vi "Main v1.1.vi"() -> ()   [LabVIEW 2017]
doc: "v0.85:\n- Counts for rejects and total\n\nv0.5:\n\n- Added Reject to Manual Mode\n- Send reject pallet cluster during manual mode\n- Run continuous manual happens only when no error has occured"
uses:
  Controls/Main Tabs v0.1.ctl
  Controls/Auto.ctl
  RT/Controls/Auto Delays.ctl
  RT/Controls/Auto Times.ctl
  support/Controls/General Para.ctl
  Controls/UI Data.ctl
  support/Controls/Auto Stats.ctl
  Controls/Logging FGV.ctl
  support/Message Queue/Enqueue Message (Single).vi
  GV/Maintenance GV.vi
  <vilib>/Utility/error.llb/Error Cluster From Error Code.vi
  <vilib>/ErrorRing/Error Ring.xnode
  support/Message Queue/Message Queue.lvlib
  support/User Event - Stop/User Event - Stop.lvlib
panel:
  in  "General Para 2":T1={"Max. Cons."=5.0, "Offset 1"=0.0, "Offset 2"=0.0, "Offset 3"=0.0, "Offset 4"=0.0} caption="General Para"
  in  "Auto Para 2":T2={"Agitator Delays"=[250, 350], "TF Delays"=[700, 800, 2], "Insertion Delays"=[100, 500], "Cutting Delays"=[300, 300, 100], "PF Delays"=[250, 30000], "Measur. Delays"=[500.0, 188.9, 1.0], "Reject Delays"=[500], "BF Delays"=[1000, 1000]}
  out "Shutdown?":bool
  out "Boolean 8":bool
  out "Boolean 7":bool
  out "Boolean 6":bool
  out "Boolean 5":bool
  out "Boolean 4":bool
  out "Boolean 3":bool
  out "Boolean 2":bool
  out "Boolean":bool
  in  "Reject Pallets":T3
  out "Date-Time":string caption="Dip-Tube Assembly Automation (HMI) v1.1"
  out "Main Tab":T4
  in  "All IOs":bool
  in  "Autocycle":T5
  in  "Manual":bool
  in  "Parameters":bool
  in  "Maintenance":bool
  in  "General Para":T1={"Max. Cons."=5.0, "Offset 1"=0.0, "Offset 2"=0.0, "Offset 3"=0.0, "Offset 4"=0.0}
  in  "BF Para":cluster{"Delay 1":u32, "Delay 2":u32}={"Delay 1"=1000, "Delay 2"=1000}
  in  "Reject Para":cluster{"Delay":u32}={"Delay"=400}
  in  "Meas. Para":T6={"Delay"=500.0, "Mean Length"=188.9, "Tolerance"=1.0}
  in  "PF Para":cluster{"Delay":u32, "Timeout":u32}={"Delay"=1000, "Timeout"=1000}
  in  "Tube Feeder Para":T7={"Delay"=400, "Delay 2"=250, "Max Attempts"=250}
  in  "Cutting Para":T8={"Delay"=400, "Delay 2"=250, "Delay 3"=250}
  in  "Agitator Para":cluster{"Delay":u32, "Timeout":u32}={"Delay"=400, "Timeout"=250}
  in  "Insertion Para":cluster{"Delay 1":u32, "Delay 2":u32}={"Delay 1"=1000, "Delay 2"=1000}
  in  "Save Para":bool
  in  "Home Para":bool
  out "OEE":dbl format="%#.1f"
  out "QUA":dbl=100.0 min=0.0 max=100.0 step=0.1
  in  "Ideal Time":dbl=2.0 min=0.0 max=100.0 step=0.1
  in  "AVL":dbl=100.0 min=0.0 max=100.0 step=0.1
  out "Rejects 2":u32 caption="Rejects"
  in  "Reset MCount":bool
  in  "Enable BF?":bool
  in  "Enable Agitate?":bool
  in  "Enable Reject?":bool
  in  "Toggle Motor":bool
  in  "Continuous?":bool
  in  "Enable Measure?":bool
  in  "Enable Index?":bool
  in  "Enable PF?":bool
  in  "Manual Para":T2={"Agitator Delays"=[400, 250], "TF Delays"=[700, 800, 2], "Insertion Delays"=[100, 500], "Cutting Delays"=[300, 300, 100], "PF Delays"=[250, 30000], "Measur. Delays"=[500.0, 188.9, 1.0], "Reject Delays"=[500], "BF Delays"=[1000, 1000]}
  in  "Enable Cutting?":bool
  in  "Enable Insertion?":bool
  in  "Run Manual":bool
  in  "Enable TF?":bool
  in  "Home Manual":bool
  out "Status 2":T10
  out "Measurements":T11 {"Height 1" format="%#.2f"; "Height 2" format="%#.2f"; "Height 3" format="%#.2f"; "Height 4" format="%#.2f"}
  out "Output Count":u32 caption="Output\nCount"
  out "PRF":dbl=100.0 min=0.0 max=100.0 step=0.1
  in  "End Cycle":bool
  out "Statuses":string[][](table)
  in  "All IO":bool
  in  "Stats":bool
  in  "Home AC":bool
  out "Status":string
  out "Count":u32 format="%06.0f"
  out "Cycle Time":dbl format="%0.2f"
  out "Rejects":u32 format="%06.0f"
  out "Output Chart":T12(graph)
  out "Reject Count":u32
  out "Total Count":u32 caption="Good Count"
  out "Total Time":dbl caption="Total Effective Cycle Time (s)" format="%#.3f"
  out "Time Chart":T13(graph)
  out "OEE Chart":T14(graph)
  out "Measurement Chart":cluster{"1":dbl, "2":dbl, "3":dbl, "4":dbl}(graph)
  out "Timestamp":string caption="Date & Timestamp"
  out "Latest Measure.":T15 caption="Latest Measurements" {"Length 1 (mm)" format="%#.2f"}
  out "Auto Times":T9
  in  "Back Stats":bool
  out "OEE 2":T14 caption="Latest Measurements" {"AVL" format="%#.1f"; "PRF" format="%#.1f"; "QUA" format="%#.1f"; "OEE" format="%#.1f"}
  in  "Home IOs":bool
  in  "Back IO":bool
  out "IAS 4":dbl format="%#.3f"
  out "IAS 3":dbl format="%#.3f"
  out "IAS 2":dbl format="%#.3f"
  out "IAS 1":dbl format="%#.3f"
  out "DI 1":T16
  out "DI 2":T17
  out "DO 1":T18
  in  "Exit":bool
  in  "Shutdown":bool
  # "HARMONY VISION DIP-TUBE ASSEMBLY AUTOMATION"
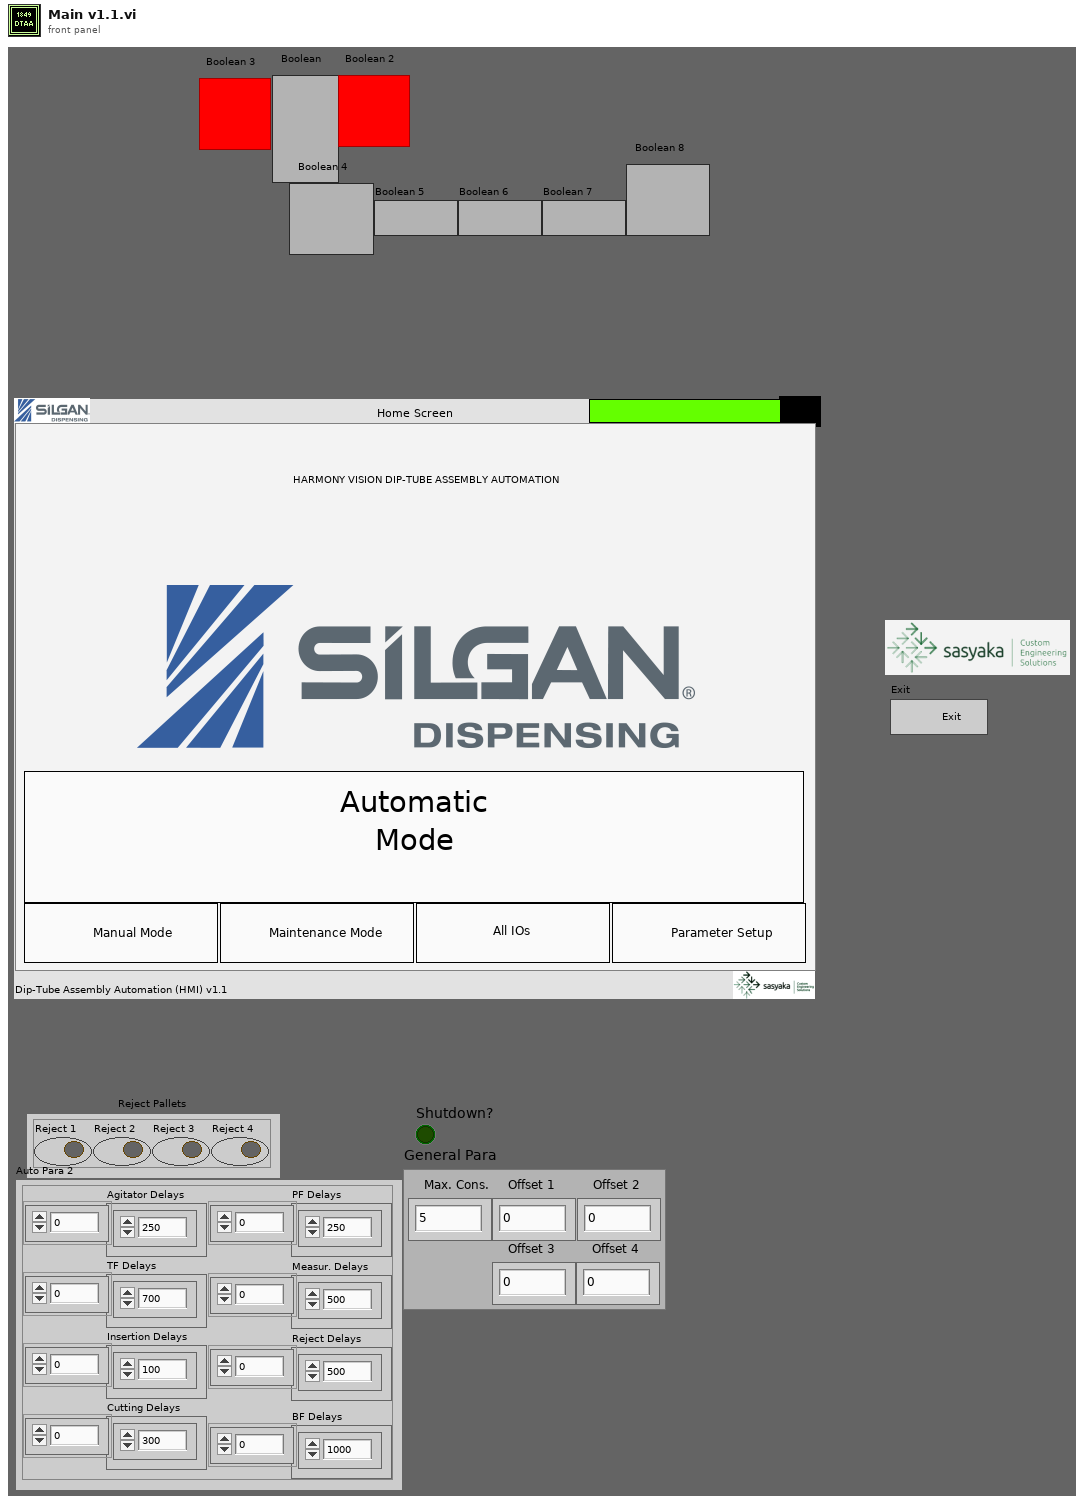
[diagram p1: front panel]
types:
  T1 = typedef "General Para.ctl" = cluster{"Max. Cons.":dbl, "Offset 1":dbl, "Offset 2":dbl, "Offset 3":dbl, "Offset 4":dbl}
  T2 = typedef "Auto Delays.ctl" = cluster{"Agitator Delays":u32[], "TF Delays":u32[], "Insertion Delays":u32[], "Cutting Delays":u32[], "PF Delays":u32[], "Measur. Delays":dbl[], "Reject Delays":u32[], "BF Delays":u32[]}
  T3 = cluster{"Reject 1":bool, "Reject 2":bool, "Reject 3":bool, "Reject 4":bool}
  T4 = typedef "Main Tabs v0.1.ctl" = enum32{"Home Screen", "Parameter Setup", "Manual Mode", "Autocycle", "Autocycle Statistics", "Autocycle IOs"}
  T5 = typedef "Auto.ctl" = bool
  T6 = cluster{"Delay":dbl, "Mean Length":dbl, "Tolerance":dbl}
  T7 = cluster{"Delay":u32, "Delay 2":u32, "Max Attempts":u32}
  T8 = cluster{"Delay":u32, "Delay 2":u32, "Delay 3":u32}
  T9 = typedef "Auto Times.ctl" = cluster{"Index Time":u32, "TF Time":u32, "Insertion Time":u32, "Cutting Time":u32, "PF Time":u32, "Meas. Time":u32, "Reject Time":u32}
  T10 = cluster{"Auto Times":T9, "error out":errorcluster}
  T11 = cluster{"Height 1":dbl, "Height 2":dbl, "Height 3":dbl, "Height 4":dbl}
  T12 = cluster{"OutputCount":u32, "Numeric Control":u32}
  T13 = cluster{"Index":dbl, "TF":dbl, "Insert":dbl, "Cutting":dbl, "PF":dbl, "Measure.":dbl, "Reject":dbl}
  T14 = cluster{"AVL":dbl, "PRF":dbl, "QUA":dbl, "OEE":dbl}
  T15 = cluster{"Length 1 (mm)":dbl, "Pallet 2 (mm)":dbl, "Pallet 3 (mm)":dbl, "Pallet 4 (mm)":dbl}
  T16 = cluster{"Machine_ON":bool, "E_stop ":bool, "SW_Pressure":bool, "SW_Start ":bool, "SW_Reset":bool, "SW_Stop":bool, "SW_Door":bool, "RS_Index_Rotary_CW":bool, "RS_Index_Rotary_CCW":bool, "RS_Index_Stopper _Rear":bool, "RS_Index_Output_Separator_Rear":bool, "PES_Index_Pallet_Sensor":bool, "PES_Index_Output_Part Sensor":bool, "ICS_BF_Low_Level_1":bool, "ICS_BF_Low_Level_2":bool, "ICS_BF_Pump_CNVR_Full_1":bool, "ICS_BF_Pump_CNVR_Full_2":bool, "ICS_BF_Pump_CNVR_Full_3":bool, "ICS_BF_Pump_CNVR_Full_4":bool, "PES_PC_Pump Presence_1":bool, "PES_PC_Pump Presence_2":bool, "PES_PC_Pump Presence_3":bool, "PES_PC_Pump Presence_4":bool, "RS_PC_Gating_Front":bool, "PES_Pump_Interference":bool, "PES_TF_Low_Level":bool, "PES_Tube Presence_1":bool, "PES_Tube Presence_2":bool, "PES_Tube Presence_3":bool, "PES_Tube Presence_4":bool, "DI1.30":bool, "DI1.31":bool}
  T17 = cluster{"RS_Agitatator_1_Rear ":bool, "RS_Agitatator_2_Rear ":bool, "RS_TF_Gating CYL_Rear":bool, "RS_Insertion_1_Rear":bool, "RS_Insertion_1_Front":bool, "RS_Insertion _2_Rear":bool, "RS_Insertion _2_Front":bool, "RS_Insertion _3_Rear":bool, "RS_Insertion _3_Front":bool, "RS_Insertion _4_Rear":bool, "RS_Insertion _4_Front":bool, "RS_Insertion_Clamp_Rear":bool, "RS_Cutting_Rear":bool, "RS_Cutting_Clamp _Rear":bool, "RS_Measurement_1_Rear":bool, "RS_Measurement_2_Rear":bool, "RS_Measurement_3_Rear":bool, "RS_Measurement_4_Rear":bool, "DI2.18":bool, "RS_Rejection_1_Rear":bool, "RS_Rejection_2_Rear":bool, "RS_Rejection_3_Rear":bool, "RS_Rejection_4_Rear":bool, "DI2.23":bool, "DI2.24":bool, "DI2.25":bool, "DI2.26":bool, "DI2.27":bool, "DI2.28":bool, "DI2.29":bool, "DI2.30":bool, "DI2.31":bool}
  T18 = cluster{"TL_Red":bool, "TL_Orange":bool, "TL_Green":bool, "TL_Buzzer":bool, "SOL_Index_Rotary_CW":bool, "SOL_Index_Rotary_CCW":bool, "SOL_Index_Stopper_Rear":bool, "SOL_OutputSeparator_Rear":bool, "Bowl  Feeder_ ON 1":bool, "Pump_CNVR_Motor _ON":bool, "SOL_PC_Gating_CYL_Rear":bool, "SOL_Tube_Feed_Agitatator":bool, "SOL_Tube_Feed_Gating_CYL":bool, "SOL_Insertion _CYL":bool, "SOL_Insertion_Clamp_CYL":bool, "SOL_Cutting_CYL":bool, "SOL_Cutting_Clamp_CYL":bool, "SOL_Insertion_Air_Nozzle":bool, "SOL_Measurement_CYL":bool, "DO1.19":bool, "SOL_Rejection CYL_1":bool, "SOL_Rejection CYL_2":bool, "SOL_Rejection CYL_3":bool, "SOL_Rejection CYL_4":bool, "Bowl  Feeder_ ON 2":bool, "SOL_BF_BlowerON":bool, "SOL_BF1_Track1":bool, "SOL_BF1_Track2":bool, "SOL_BF2_Track1":bool, "SOL_BF2_Track2":bool, "DO1.30":bool, "DO1.31":bool}
  T19 = typedef "UI Data.ctl" = cluster{"Main Tab":refnum<vi>}
  T20 = typedef "Message Queue.lvlib/All Message Queues.ctl" = cluster{"UI":refnum<queue>}
  T21 = enum8{"Enabled", "Disabled", "Disabled and Grayed Out"}
  T22 = cluster{"Array":string[][], "Machine Status":string}
  T23 = typedef "Logging FGV.ctl" = enum16{"Start Shift", "Log Index", "Read Shift", "Close Shift"}
  T24 = typedef "Auto Stats.ctl" = cluster{"Time-Stamp":timestamp, "Auto Times":T9, "Measurements":cluster{"1":dbl, "2":dbl, "3":dbl, "4":dbl}, "Outputs":cluster{"Good Parts":u32, "Reject Parts":u32}, "Cycle Time":dbl, "Remarks":string}
  T25 = cluster{"Auto Times":T9, "Results":cluster{"Measurements":cluster{"1":dbl, "2":dbl, "3":dbl, "4":dbl}, "Reject Pallets":cluster{"Reject 1":bool, "Reject 2":bool, "Reject 3":bool, "Reject 4":bool}}, "OutputCount":u32, "error out":errorcluster}
  T26 = enum8{"Information", "Error", "Successful", "Tips"}
  T27 = cluster{"Agitator Delays[0]":u32, "Agitator Delays[1]":u32}
  T28 = cluster{"TF Delays[0]":u32, "TF Delays[1]":u32, "TF Delays[2]":u32}
  T29 = cluster{"Insertion Delays[0]":u32, "Insertion Delays[1]":u32}
  T30 = cluster{"Cutting Delays[0]":u32, "Cutting Delays[1]":u32, "Cutting Delays[2]":u32}
  T31 = cluster{"Measur. Delays[0]":dbl, "Measur. Delays[1]":dbl, "Measur. Delays[2]":dbl}
  T32 = typedef "All Inputs.ctl" = cluster{"DI 1":cluster{"Machine_ON":bool, "E_stop ":bool, "SW_Pressure":bool, "SW_Start ":bool, "SW_Reset":bool, "SW_Stop":bool, "SW_Door":bool, "RS_Index_Rotary_CW":bool, "RS_Index_Rotary_CCW":bool, "RS_Index_Stopper _Rear":bool, "RS_Index_Output_Separator_Rear":bool, "PES_Index_Pallet_Sensor":bool, "PES_Index_Output_Part Sensor":bool, "ICS_BF_Low_Level_1":bool, "ICS_BF_Low_Level_2":bool, "ICS_BF_Pump_CNVR_Full_1":bool, "ICS_BF_Pump_CNVR_Full_2":bool, "ICS_BF_Pump_CNVR_Full_3":bool, "ICS_BF_Pump_CNVR_Full_4":bool, "PES_PC_Pump Presence_1":bool, "PES_PC_Pump Presence_2":bool, "PES_PC_Pump Presence_3":bool, "PES_PC_Pump Presence_4":bool, "RS_PC_Gating_Front":bool, "PES_Pump_Interference":bool, "PES_TF_Low_Level":bool, "PES_Tube Presence_1":bool, "PES_Tube Presence_2":bool, "PES_Tube Presence_3":bool, "PES_Tube Presence_4":bool, "DI1.30":bool, "DI1.31":bool}, "DI 2":cluster{"RS_Agitatator_1_Rear ":bool, "RS_Agitatator_2_Rear ":bool, "RS_TF_Gating CYL_Rear":bool, "RS_Insertion_1_Rear":bool, "RS_Insertion_1_Front":bool, "RS_Insertion _2_Rear":bool, "RS_Insertion _2_Front":bool, "RS_Insertion _3_Rear":bool, "RS_Insertion _3_Front":bool, "RS_Insertion _4_Rear":bool, "RS_Insertion _4_Front":bool, "RS_Insertion_Clamp_Rear":bool, "RS_Cutting_Rear":bool, "RS_Cutting_Clamp _Rear":bool, "RS_Measurement_1_Rear":bool, "RS_Measurement_2_Rear":bool, "RS_Measurement_3_Rear":bool, "RS_Measurement_4_Rear":bool, "RS_Measure_Clamp_Rear":bool, "RS_Rejection_1_Rear":bool, "RS_Rejection_2_Rear":bool, "RS_Rejection_3_Rear":bool, "RS_Rejection_4_Rear":bool, "DI2.23":bool, "DI2.24":bool, "DI2.25":bool, "DI2.26":bool, "DI2.27":bool, "DI2.28":bool, "DI2.29":bool, "DI2.30":bool, "DI2.31":bool}, "IAS 1":dbl, "IAS 2":dbl, "IAS 3":dbl, "IAS 4":dbl, "DO 1":cluster{"TL_Red":bool, "TL_Orange":bool, "TL_Green":bool, "TL_Buzzer":bool, "SOL_Index_Rotary_CW":bool, "SOL_Index_CNVR_Rotary_CCW":bool, "SOL_Index_CNVR_Stopper_Rear":bool, "SOL_Index_CNVR_Output _Separator _Rear":bool, "Bowl  Feeder_ ON 1":bool, "Pump_CNVR_Motor _ON":bool, "SOL_PC_Gating_CYL_Rear":bool, "SOL_Tube_Feed_Agitatator":bool, "SOL_Tube_Feed_Gating_CYL":bool, "SOL_Insertion _CYL":bool, "SOL_Insertion_Clamp_CYL":bool, "SOL_Cutting_CYL":bool, "SOL_Cutting_Clamp_CYL":bool, "SOL_Insertion_Air_Nozzle":bool, "SOL_Measurement_CYL":bool, "DO1.19":bool, "SOL_Rejection CYL_1":bool, "SOL_Rejection CYL_2":bool, "SOL_Rejection CYL_3":bool, "SOL_Rejection CYL_4":bool, "Bowl  Feeder_ ON 2":bool, "SOL_BF_BlowerON":bool, "SOL_BF1_Track1":bool, "SOL_BF1_Track2":bool, "SOL_BF2_Track1":bool, "SOL_BF2_Track2":bool, "DO1.30":bool, "DO1.31":bool}}
  T33 = cluster{"RS_Agitatator_1_Rear ":bool, "RS_Agitatator_2_Rear ":bool, "RS_TF_Gating CYL_Rear":bool, "RS_Insertion_1_Rear":bool, "RS_Insertion_1_Front":bool, "RS_Insertion _2_Rear":bool, "RS_Insertion _2_Front":bool, "RS_Insertion _3_Rear":bool, "RS_Insertion _3_Front":bool, "RS_Insertion _4_Rear":bool, "RS_Insertion _4_Front":bool, "RS_Insertion_Clamp_Rear":bool, "RS_Cutting_Rear":bool, "RS_Cutting_Clamp _Rear":bool, "RS_Measurement_1_Rear":bool, "RS_Measurement_2_Rear":bool, "RS_Measurement_3_Rear":bool, "RS_Measurement_4_Rear":bool, "RS_Measure_Clamp_Rear":bool, "RS_Rejection_1_Rear":bool, "RS_Rejection_2_Rear":bool, "RS_Rejection_3_Rear":bool, "RS_Rejection_4_Rear":bool, "DI2.23":bool, "DI2.24":bool, "DI2.25":bool, "DI2.26":bool, "DI2.27":bool, "DI2.28":bool, "DI2.29":bool, "DI2.30":bool, "DI2.31":bool}
  T34 = cluster{"TL_Red":bool, "TL_Orange":bool, "TL_Green":bool, "TL_Buzzer":bool, "SOL_Index_Rotary_CW":bool, "SOL_Index_CNVR_Rotary_CCW":bool, "SOL_Index_CNVR_Stopper_Rear":bool, "SOL_Index_CNVR_Output _Separator _Rear":bool, "Bowl  Feeder_ ON 1":bool, "Pump_CNVR_Motor _ON":bool, "SOL_PC_Gating_CYL_Rear":bool, "SOL_Tube_Feed_Agitatator":bool, "SOL_Tube_Feed_Gating_CYL":bool, "SOL_Insertion _CYL":bool, "SOL_Insertion_Clamp_CYL":bool, "SOL_Cutting_CYL":bool, "SOL_Cutting_Clamp_CYL":bool, "SOL_Insertion_Air_Nozzle":bool, "SOL_Measurement_CYL":bool, "DO1.19":bool, "SOL_Rejection CYL_1":bool, "SOL_Rejection CYL_2":bool, "SOL_Rejection CYL_3":bool, "SOL_Rejection CYL_4":bool, "Bowl  Feeder_ ON 2":bool, "SOL_BF_BlowerON":bool, "SOL_BF1_Track1":bool, "SOL_BF1_Track2":bool, "SOL_BF2_Track1":bool, "SOL_BF2_Track2":bool, "DO1.30":bool, "DO1.31":bool}
  T35 = cluster{"Manual Para":T2, "Reject Pallets":cluster{"Reject 1":bool, "Reject 2":bool, "Reject 3":bool, "Reject 4":bool}}
  T36 = cluster{"Measurements":cluster{"1":dbl, "2":dbl, "3":dbl, "4":dbl}, "Reject Pallets":cluster{"Reject 1":bool, "Reject 2":bool, "Reject 3":bool, "Reject 4":bool}}
  T37 = cluster{"Reject Pallets":cluster{"Reject 1":bool, "Reject 2":bool, "Reject 3":bool, "Reject 4":bool}, "Measurements":cluster{"1":dbl, "2":dbl, "3":dbl, "4":dbl}}
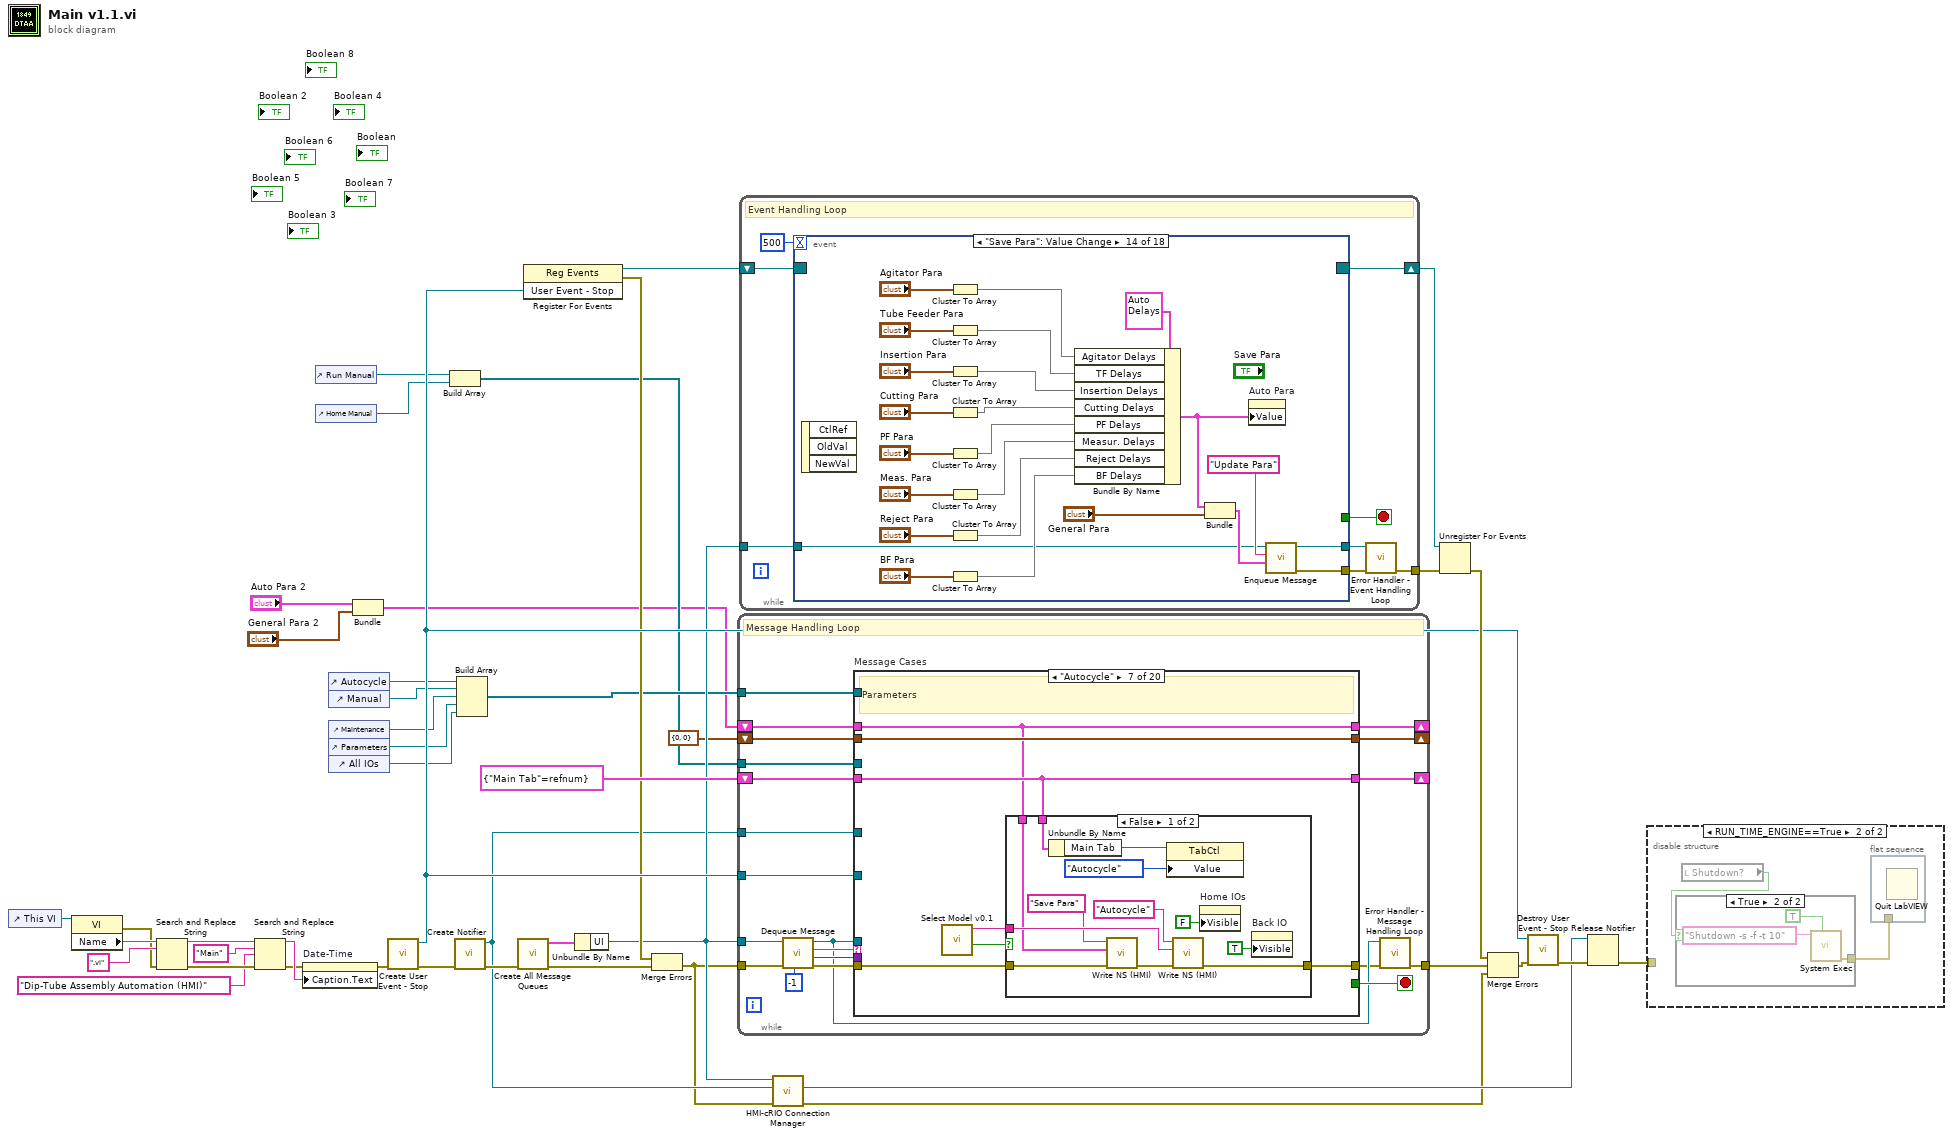
[diagram p0: block diagram]
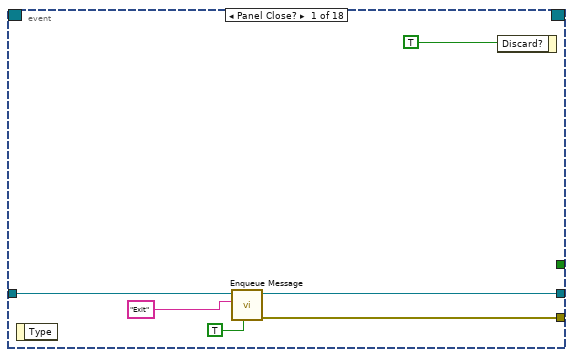
[diagram p2: hidden frame]
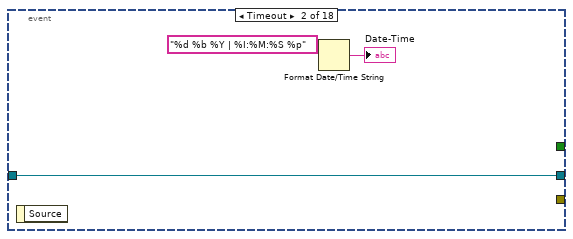
[diagram p3: hidden frame]
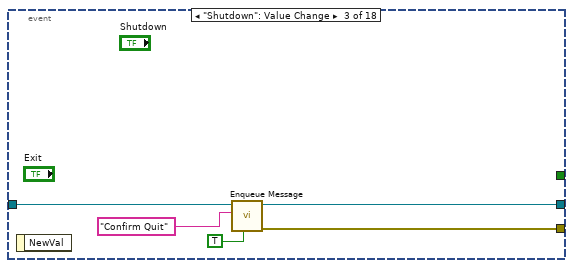
[diagram p4: hidden frame]
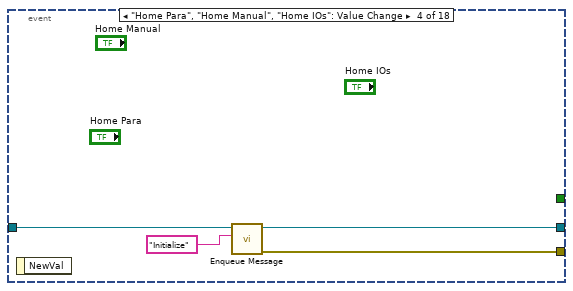
[diagram p5: hidden frame]
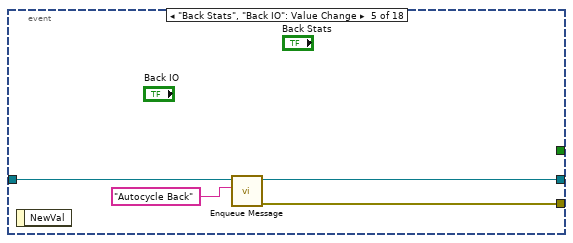
[diagram p6: hidden frame]
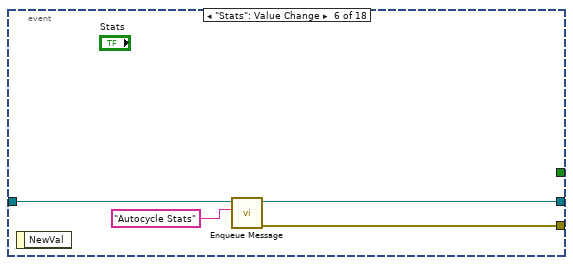
[diagram p7: hidden frame]
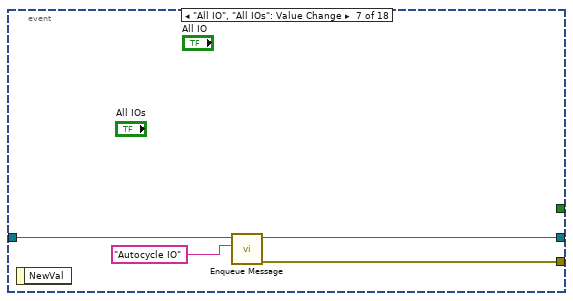
[diagram p8: hidden frame]
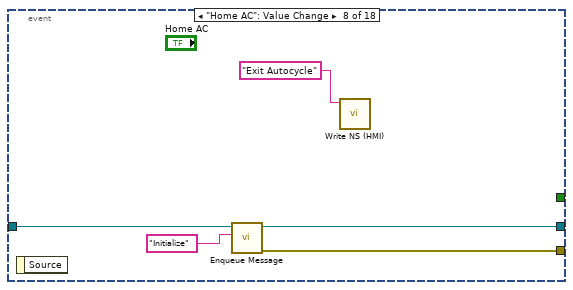
[diagram p9: hidden frame]
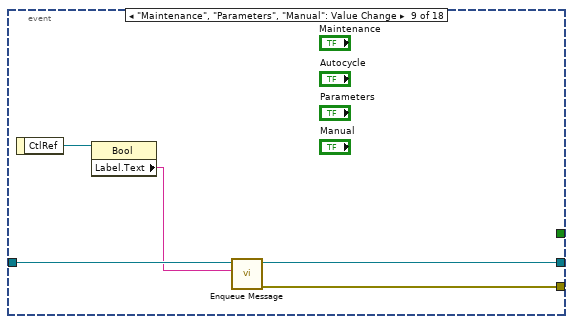
[diagram p10: hidden frame]
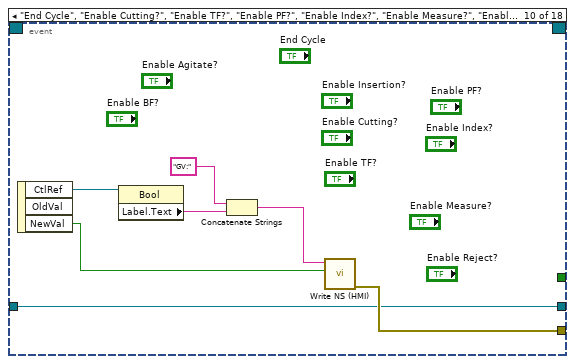
[diagram p11: hidden frame]
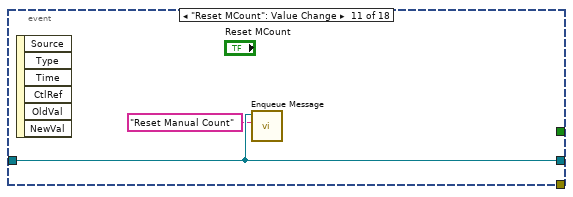
[diagram p12: hidden frame]
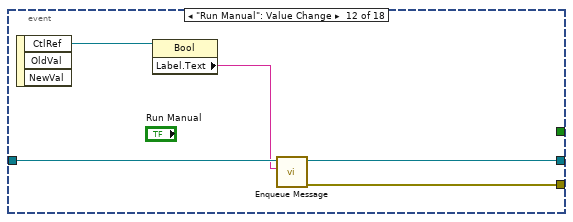
[diagram p13: hidden frame]
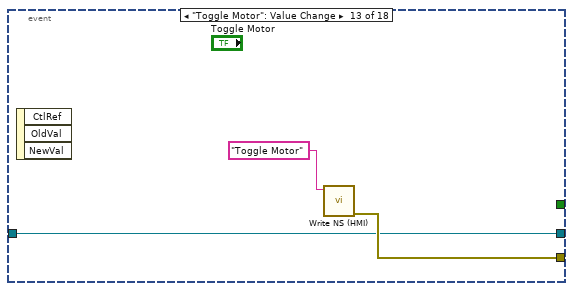
[diagram p14: hidden frame]
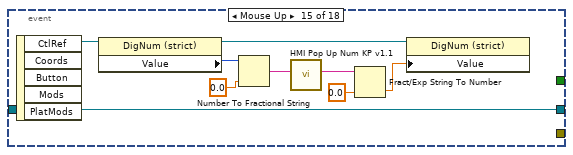
[diagram p15: hidden frame]
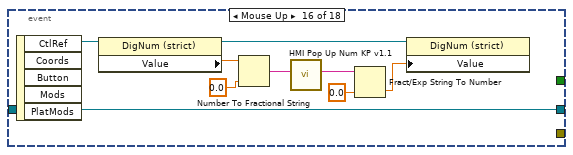
[diagram p16: hidden frame]
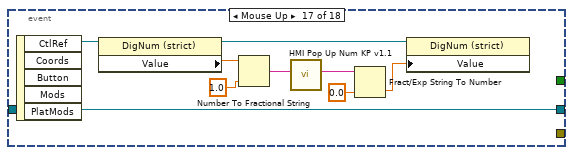
[diagram p17: hidden frame]
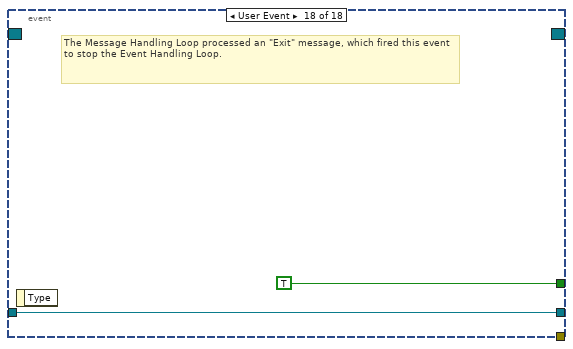
[diagram p18: hidden frame]
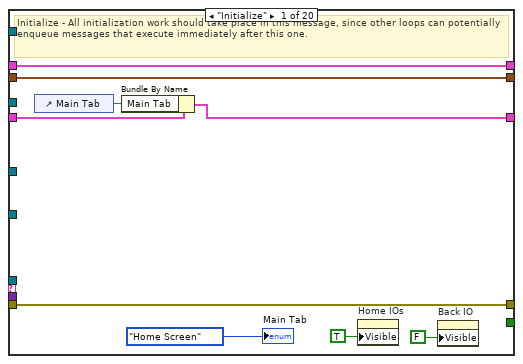
[diagram p19: hidden frame]
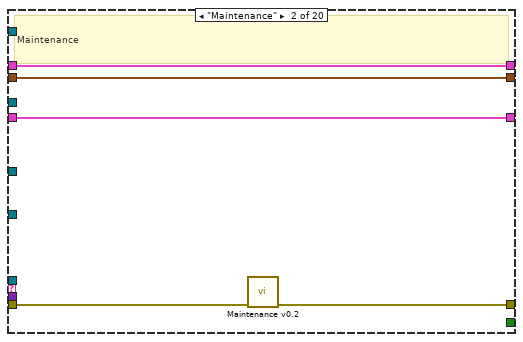
[diagram p20: hidden frame]
diagram:
  n1 = control-ref of="This VI"() -> (w15:refnum<vi>)
  n2 = property class="VI"(reference=w15) -> (error out=w14:errorcluster, "Name"=w21:string)  [unwired: 1 in, 1 out]
  n3 = Search and Replace String(input string=w21, search string=".vi", error in=w14) -> (result string=w19:string, error out=w18:errorcluster)  [unwired: 5 in, 2 out]
  n4 = Search and Replace String(input string=w19, search string="Main", replace string="Dip-Tube Assembly Automation (HMI)" ("replace string (\"\")"), error in=w18) -> (result string=w13:string, error out=w12:errorcluster)  [unwired: 4 in, 2 out]
  n5 = property on="Date-Time" class="Str"(error in=w12, "Caption.Text"=w13) -> (error out=w11:errorcluster)  [unwired: 1 in, 1 out]
  n6 = control-ref of="Run Manual"() -> (w10:refnum<vi>)
  n7 = control-ref of="Home Manual"() -> (w9:refnum<vi>)
  n8 = control-ref of="Autocycle"() -> (w26:refnum<vi>)
  n9 = control-ref of="Manual"() -> (w25:refnum<vi>)
  n10 = control-ref of="Maintenance"() -> (w24:refnum<vi>)
  n11 = control-ref of="Parameters"() -> (w23:refnum<vi>)
  n12 = control-ref of="All IOs"() -> (w4:refnum<vi>)
  n13 = Bundle("Auto Para 2"="Auto Para 2", "General Para 2"="General Para 2") -> (w1:cluster{"Auto Para 2":T2, "General Para 2":T1})  [unwired: 1 in]
  n14 = call "Create User Event - Stop.vi"("error in (no error)"=w11) -> ("error out"=w32:errorcluster, "User Event - Stop"=w35:refnum<user-event>)  [unwired: 9 in]
  n15 = Build Array(w10, w9) -> (w8:refnum<vi>[])
  n16 = call "Create Notifier.vi"("error in (no error)"=w32) -> ("error out"=w31:errorcluster, "notifier out"=w6:refnum<notifier>)  [unwired: 9 in]
  n17 = Build Array(w26, w25, w24, w23, w4) -> (w22:refnum<vi>[])
  n18 = call "Create All Message Queues.vi"("error in (no error)"=w31) -> ("error out"=w44:errorcluster, "Message Queues out"=w43:T20)  [unwired: 9 in]
  n19 = register-events(w35) -> (reference out=w36:refnum<event-registration>, error out=w34:errorcluster)  [unwired: 2 in]
  n20 = Unbundle By Name(w43) -> ("UI"=w33:refnum<queue>)
  n21 = Merge Errors(w34, w44) -> (w5:errorcluster)
  n22 = while {
    tunnel: w33 -> [w57]
    shift-right: [w64] -> _
    shift-left: T19 {"Main Tab"=refnum} ("Data Cluster") -> [w47]
    tunnel: w35 -> [w62]
    tunnel: w5 -> [w61]
    tunnel: [w55] -> w42
    tunnel: w6 -> [w52]
    tunnel: w22 -> [w51]
    tunnel: w8 -> [w50]
    shift-right: [w48] -> _
    shift-left: cluster{"OutputCount":u32, "RejectCount":u32} {"OutputCount"=0, "RejectCount"=0} -> [w49]
    shift-right: [w45] -> _
    shift-left: w1 -> [w46]
    stop <- w63 stop-if-true
    # "Message Handling Loop"
    n23 = call "Dequeue Message.vi"("timeout"=-1, "error in (no error)"=w61, "Message Queue"=w57) -> ("error out"=w60:errorcluster, "Message Data"=w58:variant, "Message"=w59:string, "dup Message Queue"=w56:refnum<queue>)  [unwired: 5 in]
    n24 = case "Message Cases" shown="\"Autocycle\"" w59 {
      selector: w59 -> [_ _ _ _ _ _ _ _ _ _ _ _ _ _ _ _ _ _ _ w362]
      tunnel: w56 -> [_ _ _ _ _ _ _ _ _ w177 w186 _ _ _ w281 _ _ w333 w359 _]
      tunnel: w60 -> [w73 w77 w91 w115 w124 w141 w149 w165 w171 w179 w194 w223 w245 w256 w289 w300 w324 w337 w352 _]
      tunnel: [w73 w76 w90 w115 w123 w141 w148 w165 w171 w178 w193 w224 w246 w258 w280 w300 w319 w335 w355 w363] -> w54
      tunnel: w47 -> [w72 w78 w93 w119 w126 w140 w145 w169 w175 w184 w191 w225 w247 w259 w290 w299 w323 w336 w358 w364]
      tunnel: [w71 w78 w93 w119 w126 w140 w145 w169 w175 w184 w191 w225 w247 w259 w290 w299 w323 w336 w358 w364] -> w64
      tunnel: [_ _ _ _ _ _ _ _ _ _ _ _ _ _ _ _ _ _ TRUE _] -> w63
      tunnel: w58 -> [_ _ w89 _ w122 _ _ _ _ _ _ w222 w244 _ w288 _ w322 _ w349 _]
      tunnel: w62 -> [_ _ _ _ _ _ _ _ _ _ _ _ _ _ _ _ _ _ w354 _]
      tunnel: w52 -> [_ _ _ _ _ _ _ _ _ _ _ _ _ _ _ _ _ _ w348 _]
      tunnel: w51 -> [_ _ w85 _ _ _ _ _ _ _ _ _ _ _ _ _ _ _ _ _]
      tunnel: w50 -> [_ _ _ _ _ _ _ _ _ _ _ _ _ w253 w286 _ _ _ _ _]
      tunnel: w49 -> [w68 w75 w80 w116 w125 w129 w150 w166 w172 w181 w195 w220 w242 w249 w279 _ w318 w332 w345 w361]
      tunnel: [w68 w75 w80 w116 w125 w129 w150 w166 w172 w181 w195 w220 w242 w249 w274 cluster{"OutputCount":u32, "RejectCount":u32} {"OutputCount"=0, "RejectCount"=0} w318 w332 w345 w361] -> w48
      tunnel: w46 -> [w65 w74 w79 w96 _ w128 w144 w164 w170 w176 w185 w209 w226 w248 w262 w296 w301 w325 w344 w360]
      tunnel: [w65 w74 w79 w96 w120 w128 w144 w164 w170 w176 w185 w209 w226 w248 w262 w296 w301 w325 w344 w360] -> w45
      frame "Initialize" {
        # "Initialize - All initialization work should take place in this message, since other loops can potentially enqueue messages that execute immediately after this one."
        n25 = control-ref of="Main Tab"() -> (w70:refnum<vi>)
        n26 = Bundle By Name(cluster=w72, "Main Tab"=w70) -> (w71:T19)
        n27 = property on="Home IOs" class="Bool"("Visible"=TRUE) -> ()  [unwired: 2 in, 2 out]
        n28 = property on="Back IO" class="Bool"("Visible"=FALSE) -> ()  [unwired: 2 in, 2 out]
        "Main Tab" <- Main_Tabs_v0.1."Home Screen" ("Main Tab")
      }
      frame "Maintenance" {
        # "Maintenance"
        n29 = call "Maintenance v0.2.vi"("Error In"=w77) -> ("Error out"=w76:errorcluster)  [unwired: 10 in]
      }
      frame "Connection" {
        n30 = Variant To Data(error in=w91, type=FALSE, Variant=w89) -> (data=w84:bool, error out=w90:errorcluster)
        n31 = Select(t=u32 6618880 ("Text.Text Colors:BG Color"), s=w84, f=u32 16762112 ("Text.Text Colors:BG Color")) -> (s? t:f=w86:u32)
        n32 = property on="Date-Time" class="Str"("Text.BGColor"=w86) -> ()  [unwired: 2 in, 2 out]
        n33 = Select(t=T21."Enabled" ("Disabled"), s=w84, f=T21."Disabled and Grayed Out") -> (s? t:f=w82:T21)
        n34 = for {
          tunnel: w85 -> [w95] mode=indexing
          tunnel: w82 -> [w94]
          n35 = property class="Bool"(reference=w95, "DisabledEnum"=w94) -> ()  [unwired: 1 in, 2 out]
        }
      }
      frame "Parameters" {
        # "Parameters"
        n36 = Unbundle(w96) -> ("Auto Para 2"=w98:T2, "General Para 2"=w97:T1)
        n37 = Unbundle By Name(w119) -> ("Main Tab"=w118:refnum<vi>)
        n38 = property on="General Para" class="Clust (strict)"("Value"=w97) -> ()  [unwired: 2 in, 2 out]
        n39 = Unbundle(w98) -> ("Agitator Delays"=w114:u32[], "TF Delays"=w113:u32[], "Insertion Delays"=w112:u32[], "Cutting Delays"=w111:u32[], "PF Delays"=w110:u32[], "Measur. Delays"=w109:dbl[], "Reject Delays"=w108:u32[], "BF Delays"=w107:u32[])
        n40 = property class="TabCtl"(reference=w118, "Value"=Main_Tabs_v0.1."Parameter Setup" ("Main Tab")) -> ()  [unwired: 1 in, 2 out]
        n41 = Array To Cluster(array=w114) -> (cluster=w106:T27)
        n42 = Array To Cluster(array=w113) -> (cluster=w105:T28)
        n43 = Array To Cluster(array=w112) -> (cluster=w104:T29)
        n44 = Array To Cluster(array=w111) -> (cluster=w103:T30)
        n45 = Array To Cluster(array=w110) -> (cluster=w102:cluster{"PF Delays[0]":u32, "PF Delays[1]":u32})
        n46 = Array To Cluster(array=w109) -> (cluster=w101:T31)
        n47 = Array To Cluster(array=w108) -> (cluster=w100:cluster{"Reject Delays[0]":u32})
        n48 = Array To Cluster(array=w107) -> (cluster=w99:cluster{"BF Delays[0]":u32, "BF Delays[1]":u32})
        n49 = property on="Agitator Para" class="Clust (strict)"("Value"=w106) -> ()  [unwired: 2 in, 2 out]
        n50 = property on="Tube Feeder Para" class="Clust (strict)"("Value"=w105) -> ()  [unwired: 2 in, 2 out]
        n51 = property on="Insertion Para" class="Clust (strict)"("Value"=w104) -> ()  [unwired: 2 in, 2 out]
        n52 = property on="Cutting Para" class="Clust (strict)"("Value"=w103) -> ()  [unwired: 2 in, 2 out]
        n53 = property on="PF Para" class="Clust (strict)"("Value"=w102) -> ()  [unwired: 2 in, 2 out]
        n54 = property on="Meas. Para" class="Clust (strict)"("Value"=w101) -> ()  [unwired: 2 in, 2 out]
        n55 = property on="Reject Para" class="Clust (strict)"("Value"=w100) -> ()  [unwired: 2 in, 2 out]
        n56 = property on="BF Para" class="Clust (strict)"("Value"=w99) -> ()  [unwired: 2 in, 2 out]
      }
      frame "Update Para" {
        # "Parameters"
        n57 = Variant To Data(error in=w124, type=cluster{"Auto Para":T2, "General Para":T1} {"Auto Para"={"Agitator Delays"=[], "TF Delays"=[], "Insertion Delays"=[], "Cutting Delays"=[], "PF Delays"=[], "Measur. Delays"=[], "Reject Delays"=[], "BF Delays"=[]}, "General Para"={"Max. Cons."=0.0, "Offset 1"=0.0, "Offset 2"=0.0, "Offset 3"=0.0, "Offset 4"=0.0}} ("cluster"), Variant=w122) -> (data=w120:cluster{"Auto Para":T2, "General Para":T1}, error out=w123:errorcluster)
      }
      frame "Manual" {
        # "Parameters"
        n58 = control-ref of="Enable Index?"() -> (w137:refnum<vi>)
        n59 = control-ref of="Enable PF?"() -> (w136:refnum<vi>)
        n60 = control-ref of="Enable Cutting?"() -> (w135:refnum<vi>)
        n61 = control-ref of="Enable Insertion?"() -> (w134:refnum<vi>)
        n62 = control-ref of="Enable TF?"() -> (w133:refnum<vi>)
        n63 = control-ref of="Enable Measure?"() -> (w131:refnum<vi>)
        n64 = Unbundle By Name(w128) -> ("Auto Para 2"=w127:T2)
        n65 = control-ref of="Enable Reject?"() -> (w130:refnum<vi>)
        n66 = Build Array(w137, w136, w135, w134, w133, w131, w130) -> (w132:refnum<vi>[])
        n67 = property on="Auto Para" class="Clust (strict)"("Value"=w127) -> ()  [unwired: 2 in, 2 out]
        n68 = for {
          tunnel: w132 -> [w143] mode=indexing
          n69 = property class="Bool (strict)"(reference=w143, "Val(Sgnl)"=FALSE ("Value (Signaling)")) -> ()  [unwired: 1 in, 2 out]
        }
        n70 = Unbundle By Name(w140) -> ("Main Tab"=w139:refnum<vi>)
        n71 = property class="TabCtl"(reference=w139, "Value"=Main_Tabs_v0.1."Manual Mode" ("Main Tab")) -> ()  [unwired: 1 in, 2 out]
      }
      frame "Autocycle" {
        # "Parameters"
        n72 = call "Select Model v0.1.vi"() -> ("Cancel out"=w146:bool, "Model out"=w147:string)  [unwired: 9 in, 1 out]
        n73 = case shown="False" w146 {
          tunnel: w149 -> [w154 w163]
          tunnel: [w161 w163] -> w148
          tunnel: w147 -> [w160 _]
          tunnel: w145 -> [w157 _]
          tunnel: w144 -> [w151 _]
          frame False {
            n74 = Unbundle By Name(w157) -> ("Main Tab"=w159:refnum<vi>)
            n75 = call "Write NS (HMI).vi"("error in (no error)"=w154, "Message Data"=w151, "Message"="Save Para") -> ("error out"=w153:errorcluster)  [unwired: 8 in]
            n76 = property class="TabCtl"(reference=w159, "Value"=Main_Tabs_v0.1."Autocycle" ("Main Tab")) -> ()  [unwired: 1 in, 2 out]
            n77 = call "Write NS (HMI).vi"("error in (no error)"=w153, "Message Data"=w160, "Message"="Autocycle") -> ("error out"=w161:errorcluster)  [unwired: 8 in]
            n78 = property on="Home IOs" class="Bool"("Visible"=FALSE) -> ()  [unwired: 2 in, 2 out]
            n79 = property on="Back IO" class="Bool"("Visible"=TRUE) -> ()  [unwired: 2 in, 2 out]
          }
          frame True {
          }
        }
      }
      frame "Autocycle Back" {
        # "Parameters"
        n80 = Unbundle By Name(w169) -> ("Main Tab"=w168:refnum<vi>)
        n81 = property class="TabCtl"(reference=w168, "Value"=Main_Tabs_v0.1."Autocycle" ("Main Tab")) -> ()  [unwired: 1 in, 2 out]
      }
      frame "Autocycle Stats" {
        # "Parameters"
        n82 = Unbundle By Name(w175) -> ("Main Tab"=w174:refnum<vi>)
        n83 = property class="TabCtl"(reference=w174, "Value"=Main_Tabs_v0.1."Autocycle Statistics" ("Main Tab")) -> ()  [unwired: 1 in, 2 out]
      }
      frame "Autocycle IO" {
        # "Parameters"
        n84 = Unbundle By Name(w184) -> ("Main Tab"=w183:refnum<vi>)
        n85 = property class="TabCtl"(reference=w183, "Value"=Main_Tabs_v0.1."Autocycle IOs" ("Main Tab")) -> ()  [unwired: 1 in, 2 out]
        n86 = call-poly "Enqueue Message.vi"("error in (no error)"=w179, "Message"="Update IO", "Message Queue"=w177) -> ("error out"=w178:errorcluster)  [unwired: 7 in, 1 out]
      }
      frame "Update IO" {
        n87 = Unbundle By Name(w191) -> ("Main Tab"=w192:refnum<vi>)
        n88 = Wait (ms)(milliseconds to wait=u32 200) -> ()  [unwired: 1 out]
        n89 = property class="TabCtl"(reference=w192) -> ("Value"=w190:variant)  [unwired: 1 in, 2 out]
        n90 = Variant To Data(type=Main_Tabs_v0.1."Autocycle IOs" ("Main Tab"), Variant=w190) -> (data=w187:T4)  [unwired: 1 in, 1 out]
        n91 = global read "Maintenance GV.vi" "All IO"() -> (w196:T32)
        n92 = case shown="\"Autocycle IOs\"" w187 {
          tunnel: w194 -> [w204 w207]
          tunnel: [w204 w206] -> w193
          tunnel: w186 -> [_ w205]
          frame Default {
          }
          frame "Autocycle IOs" {
            n93 = call-poly "Enqueue Message.vi"("error in (no error)"=w207, "Message"="Update IO", "Message Queue"=w205) -> ("error out"=w206:errorcluster)  [unwired: 7 in, 1 out]
          }
        }
        n94 = Unbundle(w196) -> ("DI 1"=→"DI 1":T16, "DI 2"=→"DI 2":T33, "IAS 1"=→"IAS 1":dbl, "IAS 2"=→"IAS 2":dbl, "IAS 3"=→"IAS 3":dbl, "IAS 4"=→"IAS 4":dbl, "DO 1"=→"DO 1":T34)
      }
      frame "Update UI" {
        # "Update Display - Convert the message data to a string to display in the Data Display indicator."
        n95 = Variant To Data(error in=w223, type=T22 {"Array"=[], "Machine Status"=""} ("Status Cluster"), Variant=w222) -> (data=w218:T22, error out=w221:errorcluster)
        n96 = Unbundle(w218) -> ("Array"=→"Statuses":string[][], "Machine Status"=w216:string)
        "Status" <- w216
        n97 = Search and Replace String(input string=w216, search string="Autocycle is Running") -> (number of replacements=w214:i32)  [unwired: 6 in, 3 out]
        n98 = Greater Than 0?(x=w214) -> (x > 0?=w212:bool)
        n99 = Select(t=T21."Disabled and Grayed Out" ("Disabled"), s=w212, f=T21."Enabled" ("Disabled")) -> (s? t:f=w211:T21)
        n100 = property on="Home AC" class="Bool"("DisabledEnum"=w211) -> ()  [unwired: 2 in, 2 out]
        n101 = Merge Errors(w221) -> (w224:errorcluster)
      }
      frame "Autocycle Log" {
        # "Update Display - Convert the message data to a string to display in the Data Display indicator."
        n102 = Variant To Data(error in=w245, type=T24 {"Time-Stamp"=timestamp(0 s since 1904-01-01), "Auto Times"={"Index Time"=0, "TF Time"=0, "Insertion Time"=0, "Cutting Time"=0, "PF Time"=0, "Meas. Time"=0, "Reject Time"=0}, "Measurements"={"1"=0.0, "2"=0.0, "3"=0.0, "4"=0.0}, "Outputs"={"Good Parts"=0, "Reject Parts"=0}, "Cycle Time"=0.0, "Remarks"=""} ("Auto Stats"), Variant=w244) -> (data=w240:T24, error out=w243:errorcluster)
        n103 = Unbundle By Name(w240) -> ("Time-Stamp"=w238:timestamp, "Measurements"=→"Latest Measure." →"Measurement Chart":cluster{"1":dbl, "2":dbl, "3":dbl, "4":dbl}, "Outputs"=→"Output Chart":cluster{"Good Parts":u32, "Reject Parts":u32}, "Auto Times"=→"Auto Times":T9)
        n104 = call "Stats Unbundle.vi"("State"=Logging_FGV."Log Index", "Auto Stats"=w240) -> ("Cycle Time"=→"Cycle Time" →"Total Time":dbl, "Counters"=w232:cluster{"GoodCount":u32, "RejectCount":u32}, "OEE Cluster"=→"OEE Chart" →"OEE 2":T14, "Total Times"=→"Time Chart":T13)  [unwired: 5 in, 1 out]
        n105 = Unbundle By Name(w232) -> ("GoodCount"=→"Count" →"Total Count":u32, "RejectCount"=→"Rejects" →"Reject Count":u32)
        n106 = Format Date/Time String(time format string (%c)="%d-%m-%Y | %H:%M:%S%3u", seconds (now)=w238) -> (date/time string=→"Timestamp":string)  [unwired: 1 in]
        n107 = Merge Errors(w243) -> (w246:errorcluster)
      }
      frame "Run Manual" {
        # "Update Manual mode"
        n108 = Bundle("Manual Para"="Manual Para", "Reject Pallets"="Reject Pallets") -> (w250:T35)  [unwired: 1 in]
        n109 = for {
          tunnel: w253 -> [w261] mode=indexing
          tunnel: T21."Disabled and Grayed Out" ("Disabled") -> [w260]
          n110 = property class="Bool"(reference=w261, "DisabledEnum"=w260) -> ()  [unwired: 1 in, 2 out]
        }
        n111 = call "Write NS (HMI).vi"("error in (no error)"=w256, "Message Data"=w250, "Message"="Manual Run") -> ("error out"=w255:errorcluster)  [unwired: 8 in]
        n112 = Merge Errors(w255) -> (w258:errorcluster)
      }
      frame "Manual Status" {
        n113 = Variant To Data(error in=w289, type=T25 {"Auto Times"={"Index Time"=0, "TF Time"=0, "Insertion Time"=0, "Cutting Time"=0, "PF Time"=0, "Meas. Time"=0, "Reject Time"=0}, "Results"={"Measurements"={"1"=0.0, "2"=0.0, "3"=0.0, "4"=0.0}, "Reject Pallets"={"Reject 1"=FALSE, "Reject 2"=FALSE, "Reject 3"=FALSE, "Reject 4"=FALSE}}, "OutputCount"=0, "error out"={"status"=FALSE, "code"=0, "source"=""}} ("cluster"), Variant=w288) -> (data=w285:T25, error out=w280:errorcluster)
        n114 = Unbundle(w285) -> ("Auto Times"=w284:T9, "Results"=w276:T36, "OutputCount"=w275:u32, "error out"=w278:errorcluster)
        n115 = for {
          tunnel: w286 -> [w295] mode=indexing
          tunnel: T21."Enabled" ("Disabled") -> [w294]
          n116 = property class="Bool"(reference=w295, "DisabledEnum"=w294) -> ()  [unwired: 1 in, 2 out]
        }
        n117 = Unbundle(w276) -> ("Measurements"=w264:cluster{"1":dbl, "2":dbl, "3":dbl, "4":dbl}, "Reject Pallets"=w265:T3)
        "Measurements" <- w264
        n118 = Bundle("Auto Times"=w284, "error out"=w278) -> (→"Status 2":T10)  [unwired: 1 in]
        n119 = Bundle("Reject Pallets"=w265, "Measurements"=w264) -> (w263:T37)  [unwired: 1 in]
        n120 = call "Counts Update (manual).vi"("output cluster"=w263, "Desired Cycle Time (s)"="Ideal Time", "AVL"="AVL", "OutputCount"=w275, "Counts in"=w279) -> ("OEE"=w269:T14, "Counts out"=w274:cluster{"OutputCount":u32, "RejectCount":u32})  [unwired: 5 in]
        n121 = Unbundle(w269) -> ("PRF"=→"PRF":dbl, "QUA"=→"QUA":dbl, "OEE"=→"OEE":dbl)  [unwired: 1 out]
        n122 = Unbundle(w274) -> ("OutputCount"=→"Output Count":u32, "RejectCount"=→"Rejects 2":u32)
        n123 = case shown="True" "Continuous?" {
          tunnel: w281 -> [_ w293]
          tunnel: w278 -> [_ w292]
          frame False {
          }
          frame True {
            # "Run if continuous is TRUE & No Error"
            n124 = call-poly "Enqueue Message.vi"("error in (no error)"=w292, "Message"="Run Manual", "Message Queue"=w293) -> ()  [unwired: 7 in, 2 out]
          }
        }
      }
      frame "Reset Manual Count" {
        w297 = u32 0 ("Rejects")
        n125 = local write "Rejects 2"(w297) -> ()
        n126 = local write "Output Count"(w297) -> ()
      }
      frame "Error" {
        w305 = 128  # call and forget
        # "Run async so that this loop will continue to run"
        # "Error"
        n127 = Variant To Data(error in=w324, type=errorcluster {"status"=FALSE, "code"=0, "source"=""} ("error constant"), Variant=w322) -> (data=w317:errorcluster, error out=w320:errorcluster)
        n128 = Unbundle By Name(w317) -> ("source"=w316:string)
        n129 = vi-ref "NewDialog.vi"() -> (w312:refnum<vi>)
        n130 = property class="VI"(reference=w312) -> (error out=w314:errorcluster, "Name"=w313:string)  [unwired: 1 in, 1 out]
        n131 = Search and Replace String(input string=w316, search string="<err>") -> (result string=w304:string)  [unwired: 6 in, 3 out]
        n132 = Open VI Reference(type specifier VI Refnum (for type only)=refnum<vi> refnum, vi path=w313, options=w305, error in (no error)=w314) -> (vi reference=w307:refnum<vi>, error out=w308:errorcluster)  [unwired: 2 in]
        n133 = call-by-ref "Start Asynchronous Call"(reference=w307, error in=w308, "inIcon"=T26."Error", "inTitle"="ERROR", "inMessage"=w304) -> (reference out=w310:refnum<vi>, error out=w309:errorcluster)  [unwired: 6 in, 3 out]
        n134 = Close Reference(reference=w310, error in (no error)=w309) -> (error out=w311:errorcluster)
        n135 = call <vilib>:"Simple Error Handler.vi"("error in (no error)"=w311) -> ()  [unwired: 4 in, 5 out]
        n136 = Merge Errors(w320) -> (w319:errorcluster)
      }
      frame "Confirm Quit" {
        # "Confirm Quit - Message that can confirm whether or not the user wants to exit the application."
        n137 = call "NewDialog.vi"("inIcon"=T26."Information", "inTitle"="SHUTDOWN?", "inButton2Text"="Shutdown", "inButton1Text"="", "inMessage"="Are you sure you want to shutdown?") -> ("outButton2"=w326:bool)  [unwired: 4 in, 2 out]
        "Shutdown?" <- w326
        n138 = case shown="True" w326 {
          tunnel: w337 -> [w338 w343]
          tunnel: [w338 w342] -> w334
          tunnel: w333 -> [_ w341]
          frame False {
          }
          frame True {
            n139 = call-poly "Enqueue Message.vi"("Priority Message? (F)"=TRUE, "error in (no error)"=w343, "Message"="Exit", "Message Queue"=w341) -> ("error out"=w342:errorcluster)  [unwired: 6 in, 1 out]
          }
        }
        n140 = Merge Errors(w334) -> (w335:errorcluster)
      }
      frame "Exit" {
        # "Stop the VI"
        # "Release the message queue reference"
        # "Exit - Exit the application."
        n141 = Variant To Data(type=errorcluster {"status"=FALSE, "code"=0, "source"=""} ("error constant"), Variant=w349) -> (data=w350:errorcluster)  [unwired: 1 in, 1 out]
        n142 = call <vilib>:"Simple Error Handler.vi"("error in (no error)"=w350) -> ()  [unwired: 4 in, 5 out]
        n143 = Send Notification(notification=TRUE, notifier=w348) -> (error out=w346:errorcluster)  [unwired: 1 in, 1 out]
        n144 = call "Fire User Event - Stop.vi"("User Event - Stop"=w354) -> ("error out"=w353:errorcluster)  [unwired: 10 in]
        n145 = Release Queue(queue=w359, error in (no error)=w352) -> (error out=w356:errorcluster)  [unwired: 1 in, 2 out]
        n146 = Merge Errors(w346, w353, w356) -> (w355:errorcluster)
      }
      frame Default {
        # "'Default' case only runs if there is a message that isn't defined in any of the other cases.  Output a programming error."
        n147 = xnode "Error Ring"("parameter 0"=w362) -> ("error out"=w363:errorcluster)
      }
    }
    n148 = call "Error Handler - Message Handling Loop.vi"("error in (no error)"=w54, "Message Queue"=w56) -> ("dup error in"=w55:errorcluster)  [unwired: 8 in, 1 out]
  }
  n149 = while {
    tunnel: w33 -> [w379]
    shift-right: [w377] -> w39
    shift-left: w36 -> [w378]
    tunnel: [w373] -> w37
    stop <- w375 stop-if-true
    # "Event Handling Loop"
    n150 = event shown="[13] \"Save Para\": Value Change" {
      selector: w378 -> [_ _ _ _ _ _ _ _ _ _ _ _ _ _ _ _ _ _]
      dyn-events: [_ _ _ _ _ _ _ _ _ _ _ _ _ _ _ _ _ _] -> w377
      timeout: 500 -> [_ _ _ _ _ _ _ _ _ _ _ _ _ _ _ _ _ _]
      tunnel: [_ _ _ _ _ _ _ _ _ _ _ _ _ _ _ _ _ TRUE ("Discard?")] -> w375
      tunnel: w379 -> [w384 w388 w393 w397 w401 w405 w409 w414 w419 w424 w428 w433 w435 w438 w469 w478 w487 w489]
      tunnel: [w383 _ w392 w396 w400 w404 w408 w413 w418 w425 _ w431 w436 w441 _ _ _ _] -> w376
      tunnel: [w382 w388 w391 w395 w399 w403 w407 w412 w417 w424 w428 w432 w435 w437 w469 w478 w487 w489] -> w374
      event Panel Close? {
        n151 = event-data() -> ()  [unwired: 1 in, 1 out]
        n152 = call-poly "Enqueue Message.vi"("Priority Message? (F)"=TRUE, "Message"="Exit", "Message Queue"=w384) -> ("error out"=w383:errorcluster, "dup Message Queue"=w382:refnum<queue>)  [unwired: 7 in]
        n153 = event-data("Discard?"=TRUE) -> ()  [unwired: 1 in, 1 out]
      }
      event Timeout {
        n154 = event-data() -> ()  [unwired: 1 in, 1 out]
        n155 = Format Date/Time String(time format string (%c)="%d %b %Y | %I:%M:%S %p") -> (date/time string=→"Date-Time":string)  [unwired: 2 in]
      }
      event "Shutdown": Value Change {
        n156 = event-data() -> ()  [unwired: 1 in, 1 out]
        n157 = call-poly "Enqueue Message.vi"("Priority Message? (F)"=TRUE, "Message"="Confirm Quit", "Message Queue"=w393) -> ("error out"=w392:errorcluster, "dup Message Queue"=w391:refnum<queue>)  [unwired: 7 in]
      }
      event "Home Para", "Home Manual", "Home IOs": Value Change {
        n158 = event-data() -> ()  [unwired: 1 in, 1 out]
        n159 = call-poly "Enqueue Message.vi"("Message"="Initialize", "Message Queue"=w397) -> ("error out"=w396:errorcluster, "dup Message Queue"=w395:refnum<queue>)  [unwired: 8 in]
      }
      event "Back Stats", "Back IO": Value Change {
        n160 = event-data() -> ()  [unwired: 1 in, 1 out]
        n161 = call-poly "Enqueue Message.vi"("Message"="Autocycle Back", "Message Queue"=w401) -> ("error out"=w400:errorcluster, "dup Message Queue"=w399:refnum<queue>)  [unwired: 8 in]
      }
      event "Stats": Value Change {
        n162 = event-data() -> ()  [unwired: 1 in, 1 out]
        n163 = call-poly "Enqueue Message.vi"("Message"="Autocycle Stats", "Message Queue"=w405) -> ("error out"=w404:errorcluster, "dup Message Queue"=w403:refnum<queue>)  [unwired: 8 in]
      }
      event "All IO", "All IOs": Value Change {
        n164 = event-data() -> ()  [unwired: 1 in, 1 out]
        n165 = call-poly "Enqueue Message.vi"("Message"="Autocycle IO", "Message Queue"=w409) -> ("error out"=w408:errorcluster, "dup Message Queue"=w407:refnum<queue>)  [unwired: 8 in]
      }
      event "Home AC": Value Change {
        n166 = event-data() -> ()  [unwired: 1 in, 1 out]
        n167 = call-poly "Enqueue Message.vi"("Message"="Initialize", "Message Queue"=w414) -> ("error out"=w413:errorcluster, "dup Message Queue"=w412:refnum<queue>)  [unwired: 8 in]
        n168 = call "Write NS (HMI).vi"("Message"="Exit Autocycle") -> ()  [unwired: 10 in, 1 out]
      }
      event "Maintenance", "Parameters", "Manual": Value Change {
        n169 = event-data() -> ("CtlRef"=w416:refnum<vi>)  [unwired: 1 in]
        n170 = property class="Bool"(reference=w416) -> ("Label.Text"=w415:string)  [unwired: 1 in, 2 out]
        n171 = call-poly "Enqueue Message.vi"("Message"=w415, "Message Queue"=w419) -> ("error out"=w418:errorcluster, "dup Message Queue"=w417:refnum<queue>)  [unwired: 8 in]
      }
      event "End Cycle", "Enable Cutting?", "Enable TF?", "Enable PF?", "Enable Index?", "Enable Measure?", "Enable Reject?", "Enable Agitate?", "Enable BF?": Value Change {
        n172 = event-data() -> ("CtlRef"=w426:refnum<vi>, "NewVal"=w420:bool)  [unwired: 1 in, 1 out]
        n173 = property class="Bool"(reference=w426) -> ("Label.Text"=w423:string)  [unwired: 1 in, 2 out]
        n174 = Concatenate Strings("GV:" ("string"), w423) -> (w421:string)
        n175 = call "Write NS (HMI).vi"("Message Data"=w420, "Message"=w421) -> ("error out"=w425:errorcluster)  [unwired: 9 in]
      }
      event "Reset MCount": Value Change {
        n176 = event-data() -> ()  [unwired: 1 in, 6 out]
        n177 = call-poly "Enqueue Message.vi"("Message"="Reset Manual Count", "Message Queue"=w428) -> ()  [unwired: 8 in, 2 out]
      }
      event "Run Manual": Value Change {
        n178 = event-data() -> ("CtlRef"=w430:refnum<vi>)  [unwired: 1 in, 2 out]
        n179 = property class="Bool"(reference=w430) -> ("Label.Text"=w429:string)  [unwired: 1 in, 2 out]
        n180 = call-poly "Enqueue Message.vi"("Message"=w429, "Message Queue"=w433) -> ("error out"=w431:errorcluster, "dup Message Queue"=w432:refnum<queue>)  [unwired: 8 in]
      }
      event "Toggle Motor": Value Change {
        n181 = event-data() -> ()  [unwired: 1 in, 3 out]
        n182 = call "Write NS (HMI).vi"("Message"="Toggle Motor") -> ("error out"=w436:errorcluster)  [unwired: 10 in]
      }
      event "Save Para": Value Change {
        n183 = event-data() -> ()  [unwired: 1 in, 3 out]
        n184 = Cluster To Array(cluster="Agitator Para") -> (array=w458:u32[])
        n185 = Cluster To Array(cluster="Tube Feeder Para") -> (array=w456:u32[])
        n186 = Cluster To Array(cluster="Insertion Para") -> (array=w454:u32[])
        n187 = Cluster To Array(cluster="Cutting Para") -> (array=w452:u32[])
        n188 = Cluster To Array(cluster="PF Para") -> (array=w450:u32[])
        n189 = Cluster To Array(cluster="Meas. Para") -> (array=w448:dbl[])
        n190 = Cluster To Array(cluster="Reject Para") -> (array=w446:u32[])
        n191 = Cluster To Array(cluster="BF Para") -> (array=w444:u32[])
        n192 = Bundle By Name(cluster=T2 {"Agitator Delays"=[1000], "TF Delays"=[1000], "Insertion Delays"=[1000], "Cutting Delays"=[1000], "PF Delays"=[1000], "Measur. Delays"=[1000.0], "Reject Delays"=[1000], "BF Delays"=[1000]} ("Auto Para"), "Agitator Delays"=w458, "TF Delays"=w456, "Insertion Delays"=w454, "Cutting Delays"=w452, "PF Delays"=w450, "Measur. Delays"=w448, "Reject Delays"=w446, "BF Delays"=w444) -> (w443:T2)
        n193 = Bundle("Auto Para"=w443, "General Para"="General Para") -> (w440:cluster{"Auto Para":T2, "General Para":T1})  [unwired: 1 in]
        n194 = property on="Auto Para" class="Clust (strict)"("Value"=w443) -> ()  [unwired: 2 in, 2 out]
        n195 = call-poly "Enqueue Message.vi"("Message Data"=w440, "Message"="Update Para", "Message Queue"=w438) -> ("error out"=w441:errorcluster, "dup Message Queue"=w437:refnum<queue>)  [unwired: 7 in]
      }
      event "Insertion Para.Delay 1", "Insertion Para.Delay 2", "Agitator Para.Delay", "Agitator Para.Timeout", "Cutting Para.Delay", "Cutting Para.Delay 2", "Cutting Para.Delay 3", "Tube Feeder Para.Delay", "Tube Feeder Para.Delay 2", "Tube Feeder Para.Max Attempts", "PF Para.Delay", "PF Para.Timeout", "Reject Para.Delay", "BF Para.Delay 1", "BF Para.Delay 2": Mouse Up {
        n196 = event-data() -> ("CtlRef"=w461:refnum<vi>)  [unwired: 1 in, 4 out]
        n197 = property class="DigNum (strict)"(reference=w461) -> (reference out=w464:refnum<vi>, "Value"=w465:u32)  [unwired: 1 in, 1 out]
        n198 = Number To Fractional String(number=w465, precision (6)=0.0 ("width (-)")) -> (F-format string=w463:string)  [unwired: 2 in]
        n199 = call "HMI Pop Up Num KP v1.1.vi"("String In"=w463) -> ("String Out"=w462:string)  [unwired: 9 in, 1 out]
        n200 = Fract/Exp String To Number(string=w462, default (0 dbl)=0.0 ("default (0 I32)")) -> (number=w467:dbl)  [unwired: 2 in, 1 out]
        n201 = property class="DigNum (strict)"(reference=w464, "Value"=w467) -> ()  [unwired: 1 in, 2 out]
      }
      event "Meas. Para.Delay": Mouse Up {
        n202 = event-data() -> ("CtlRef"=w470:refnum<vi>)  [unwired: 1 in, 4 out]
        n203 = property class="DigNum (strict)"(reference=w470) -> (reference out=w473:refnum<vi>, "Value"=w474:dbl)  [unwired: 1 in, 1 out]
        n204 = Number To Fractional String(number=w474, precision (6)=0.0 ("width (-)")) -> (F-format string=w472:string)  [unwired: 2 in]
        n205 = call "HMI Pop Up Num KP v1.1.vi"("String In"=w472) -> ("String Out"=w471:string)  [unwired: 9 in, 1 out]
        n206 = Fract/Exp String To Number(string=w471, default (0 dbl)=0.0 ("default (0 I32)")) -> (number=w476:dbl)  [unwired: 2 in, 1 out]
        n207 = property class="DigNum (strict)"(reference=w473, "Value"=w476) -> ()  [unwired: 1 in, 2 out]
      }
      event "Meas. Para.Mean Length", "Meas. Para.Tolerance": Mouse Up {
        n208 = event-data() -> ("CtlRef"=w479:refnum<vi>)  [unwired: 1 in, 4 out]
        n209 = property class="DigNum (strict)"(reference=w479) -> (reference out=w482:refnum<vi>, "Value"=w483:dbl)  [unwired: 1 in, 1 out]
        n210 = Number To Fractional String(number=w483, precision (6)=1.0 ("width (-)")) -> (F-format string=w481:string)  [unwired: 2 in]
        n211 = call "HMI Pop Up Num KP v1.1.vi"("String In"=w481) -> ("String Out"=w480:string)  [unwired: 9 in, 1 out]
        n212 = Fract/Exp String To Number(string=w480, default (0 dbl)=0.0 ("default (0 I32)")) -> (number=w485:dbl)  [unwired: 2 in, 1 out]
        n213 = property class="DigNum (strict)"(reference=w482, "Value"=w485) -> ()  [unwired: 1 in, 2 out]
      }
      event User Event {
        # "The Message Handling Loop processed an \"Exit\" message, which fired this event to stop the Event Handling Loop."
        n214 = event-data() -> ()  [unwired: 1 in, 1 out]
      }
    }
    n215 = call "Error Handler - Event Handling Loop.vi"("error in (no error)"=w376, "Message Queue"=w374) -> ("dup error in"=w373:errorcluster)  [unwired: 8 in, 1 out]
  }
  n216 = call "HMI-cRIO Connection Manager.vi"("error in"=w5, "notifier in"=w6, "Queue in"=w33) -> ("error out"=w27:errorcluster, "Notifier out"=w28:refnum<notifier>)  [unwired: 7 in]
  n217 = Unregister For Events(event registration refnum=w39, error in=w37) -> (error out=w40:errorcluster)
  n218 = Merge Errors(w40, w42, w27) -> (w41:errorcluster)
  n219 = call "Destroy User Event - Stop.vi"("error in (no error)"=w41, "User Event - Stop"=w35) -> ("error out"=w30:errorcluster)  [unwired: 9 in]
  n220 = Release Notifier(notifier=w28, error in (no error)=w30) -> (error out=w29:errorcluster)  [unwired: 1 in, 2 out]
  n221 = disable-structure shown="RUN_TIME_ENGINE==True" {
    disable-tunnel: w29 -> [_ _]
    frame condition #0 (active) {
    }
    frame condition #1 {
      n222 = local read "Shutdown?"() -> (w490:bool)
      n223 = case shown="True" w490 {
        tunnel: [_ w492] -> w491
        frame False {
        }
        frame True {
          n224 = call <vilib>:"System Exec.vi"("wait until completion? (T)"=TRUE, "command line"="Shutdown -s -f -t 10") -> ("error out"=w492:errorcluster)  [unwired: 6 in, 3 out]
        }
      }
      n225 = flat-sequence {
        tunnel: w491 -> [_]
        frame #0 {
          n226 = Quit LabVIEW() -> ()  [unwired: 1 in]
        }
      }
    }
  }
